vi "enqueue_states.vi"(7 "task":T1=[enum."(qsm) initialize"], 8 "error in":errorcluster, 11 "queue in":refnum<queue>) -> (0 "error out":errorcluster, 3 "queue out":refnum<queue>)   [LabVIEW 2016]
uses:
  type defs/state.ctl
  type defs/task.ctl
panel:
  # "enqueue_states"
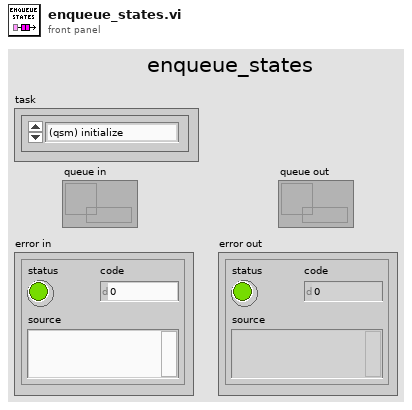
[diagram p1: front panel]
types:
  T1 = typedef "task.ctl" = T2[]
  T2 = typedef "state.ctl" = enum16{"(qsm) schedule", "(qsm) initialize", "(qsm) release", "(qsm) clean up", "(qsm) shutdown", "(myRIO) initialize", "(myRIO) clean up", "(myRIO) update ports", "(image) get", "(image) analyze", "(image) overlay", "(image) show", "save image", "state A", "state B", "state C", "state D", "state E", "state F", "state G", "state H"}
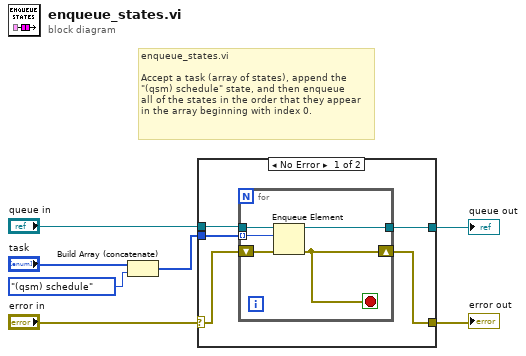
[diagram p0: block diagram]
diagram:
  # "enqueue_states.vi\n\nAccept a task (array of states), append the\n\"(qsm) schedule\" state, and then enqueue\nall of the states in the order that they appear\nin the array beginning with index 0."
  n1 = Build Array (concatenate) "Build Array"("task", state."(qsm) schedule" ("element")) -> (w2:T1)
  n2 = case shown="No Error" "error in" {
    selector: "error in" -> [w10 w19]
    tunnel: [w9 w19] -> w6
    tunnel: "queue in" -> [w12 w18]
    tunnel: [w11 w18] -> w4
    tunnel: w2 -> [w8 _]
    frame No Error {
      n3 = for {
        shift-right: [w15] -> w9
        shift-left: w10 -> [w17]
        tunnel: w12 -> [w16]
        tunnel: w8 -> [w13] mode=indexing
        tunnel: [w14] -> w11
        stop <- w15 stop-if-true
        n4 = Enqueue Element(queue=w16, element=w13, error in (no error)=w17) -> (queue out=w14:refnum<queue>, error out=w15:errorcluster)  [unwired: 1 in, 1 out]
      }
    }
    frame Error {
    }
  }
  "queue out" <- w4
  "error out" <- w6
